vi "Read Input DBL Values.vi"(8 "error in (no error)":errorcluster, 9 "number of registers":u16, 10 "starting address":u16, 11 "device data model in":refnum<class "ICPCON ET Data Model.lvclass">) -> (0 "error out":errorcluster, 2 "Values":dbl[](array[numeric]), 3 "device data model out":refnum<class "ICPCON ET Data Model.lvclass">)   [LabVIEW 2021, in "ICPCON ET Data Model.lvclass"]
doc: "Reads N input registers from the device model, starting at register M."
uses:
  ICPCON ET Data Model.lvclass
  ICPCON ET Data Model.lvclass/ICPCON ET Data Model.ctl
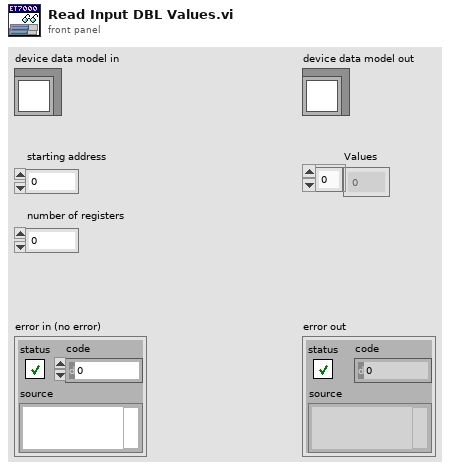
[diagram p1: front panel]
types:
  T1 = typedef "ICPCON ET Data Model.lvclass/Data Model.ctl" = cluster{"UTC":u64, "DI":bool[], "DO":bool[], "IR":u16[], "HR":u16[], "ES":u8}
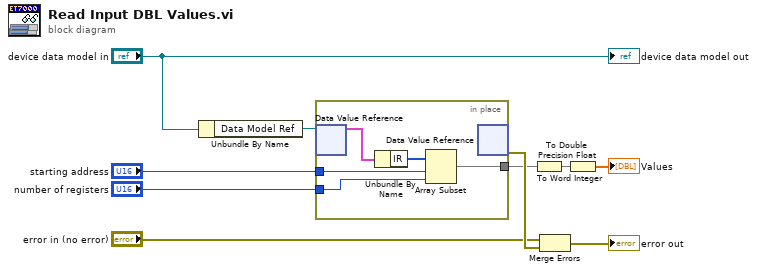
[diagram p0: block diagram]
diagram:
  n1 = Unbundle By Name("device data model in") -> ("Data Model Ref"=w6:refnum<data-value>)
  n2 = in-place {
    in-place-border: "starting address" -> [w12]
    in-place-border: "number of registers" -> [w11]
    in-place-border: [w13] -> w2
    n3 = in-place-dvr #1(w6) -> (w15:T1)  [unwired: 1 out]
    n4 = Unbundle By Name(w15) -> ("IR"=w14:u16[])
    n5 = Array Subset(array=w14, index=w12, length=w11) -> (w13:u16[])
    n6 = in-place-dvr #1() -> (w5:errorcluster)  [unwired: 1 in, 1 out]
  }
  n7 = To Word Integer(number=w2) -> (16bit integer=w3:i16[])
  n8 = Merge Errors("error in (no error)", w5) -> (→"error out":errorcluster)
  n9 = To Double Precision Float(number=w3) -> (double precision float=→"Values":dbl[])
  "device data model out" <- "device data model in"
